vi "Delete Context Menu Item.vi"(0 "NotifyIcon in":refnum<class "NotifyIcon.lvclass">, 5 "Item Tag":string, 11 "error in (no error)":errorcluster) -> (4 "NotifyIcon out":refnum<class "NotifyIcon.lvclass">, 6 "Deleted Item Tag":string, 15 "error out":errorcluster)   [LabVIEW 2016, in "NotifyIcon.lvclass"]
doc: "This VI deletes a menu item from the Context Menu. All child items and submenus are deleted and disposed of recursively.\n\n\nStinus Olsen\nCIM Industrial Systems A/S\n22. Feb. 2011 15:04\nmailto: seo@cim.as"
uses:
  NotifyIcon.lvclass
  System.Windows.Forms
panel:
  # "This VI belongs to the NotifyIcon Toolset. \nA toolset that makes it easy to create, control and manipulate a notification icon in the notification area of the Windows taskbar.\nThe toolset requires Microsoft .NET framework 2.0\n\n\nNOTICE -- YOU MUST LEAVE THIS NOTICE IN PLACE.  PER THE TERMS OF THE LICENSE BELOW, YOU MAY SUBLICENSE THIS SOFTWARE \nIN ANY WAY THAT DOES NOT CONFLICT WITH THIS LICENSE.\n\n### BSD License (http://www.opensource.org/licenses/bsd-license.php) Begin ###\n \nCopyright (c) 2011, Stinus Olsen <seo@cim.as>\n\nAll rights reserved.\n\nRedistribution and use in source and binary forms, with or without modification, are permitted provided that the following conditions are met:\n\n    * Redistributions of source code must retain the above copyright notice, this list of conditions and the following disclaimer.\n    * Redistributions in binary form must reproduce the above copyright notice, this list of conditions and the following disclaimer in the \n       documentation and/or other materials provided with the distribution.\n    * Neither the name of CIM Industrial Systems nor the names of its contributors may be used to endorse or promote products derived \n       from this software without specific prior written permission.\n\nTHIS SOFTWARE IS PROVIDED BY THE COPYRIGHT HOLDERS AND CONTRIBUTORS \"AS IS\" AND ANY EXPRESS OR IMPLIED WARRANTIES, \nINCLUDING, BUT NOT LIMITED TO, THE IMPLIED WARRANTIES OF MERCHANTABILITY AND FITNESS FOR A PARTICULAR PURPOSE ARE \nDISCLAIMED. IN NO EVENT SHALL THE COPYRIGHT OWNER OR CONTRIBUTORS BE LIABLE FOR ANY DIRECT, INDIRECT, INCIDENTAL,\n SPECIAL, EXEMPLARY, OR CONSEQUENTIAL DAMAGES (INCLUDING, BUT NOT LIMITED TO, PROCUREMENT OF SUBSTITUTE GOODS OR \nSERVICES; LOSS OF USE, DATA, OR PROFITS; OR BUSINESS INTERRUPTION) HOWEVER CAUSED AND ON ANY THEORY OF LIABILITY, \nWHETHER IN CONTRACT, STRICT LIABILITY, OR TORT (INCLUDING NEGLIGENCE OR OTHERWISE) ARISING IN ANY WAY OUT OF THE USE \nOF THIS SOFTWARE, EVEN IF ADVISED OF THE POSSIBILITY OF SUCH DAMAGE.\n\n### BSD License End ###"
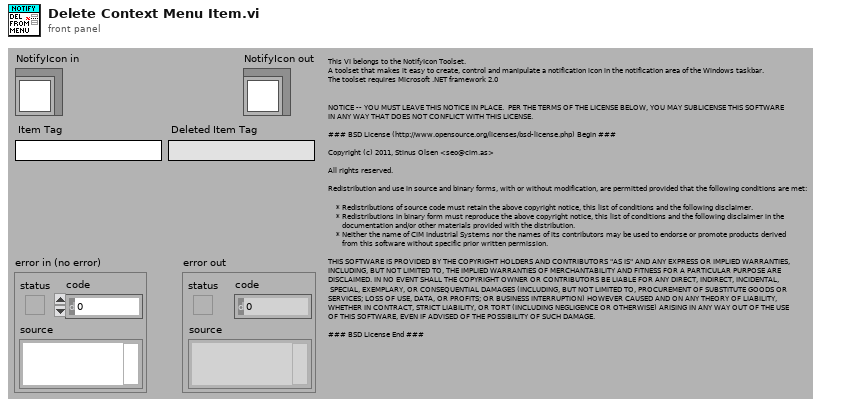
[diagram p1: front panel]
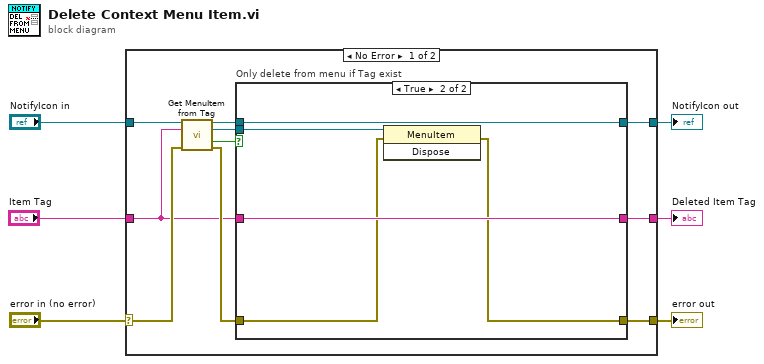
[diagram p0: block diagram]
diagram:
  n1 = case shown="No Error" "error in (no error)" {
    selector: "error in (no error)" -> [w12 w25]
    tunnel: [w15 w25] -> w5
    tunnel: [w16 w24] -> w3
    tunnel: "NotifyIcon in" -> [w14 w24]
    tunnel: "Item Tag" -> [w9 _]
    tunnel: [w8 _] -> w1
    frame No Error {
      n2 = call "Get MenuItem from Tag.vi"("NotifyIcon in"=w14, "Item Tag"=w9, "error in (no error)"=w12) -> ("NotifyIcon out"=w13:refnum<class "NotifyIcon.lvclass">, "MenuItem"=w7:refnum<k24>, "Found"=w10:bool, "error out"=w11:errorcluster)  [unwired: 9 out]
      n3 = case "Only delete from menu if Tag exist" shown="True" w10 {
        tunnel: w11 -> [w17 w21]
        tunnel: w13 -> [w18 w19]
        tunnel: [w18 w19] -> w16
        tunnel: [w17 w20] -> w15
        tunnel: [_ w23] -> w8
        tunnel: w9 -> [_ w23]
        tunnel: w7 -> [_ w22]
        frame False {
          # "Cannot delete node that is not found"
        }
        frame True {
          n4 = invoke class="MenuItem" method="Dispose"(reference=w22, error in=w21) -> (error out=w20:errorcluster)  [unwired: 1 in, 2 out]
        }
      }
    }
    frame Error {
    }
  }
  "error out" <- w5
  "NotifyIcon out" <- w3
  "Deleted Item Tag" <- w1
